vi "Launch Event Handler.vi"(8 "error in (no error)":errorcluster, 11 "Control in":refnum<class "Control.lvclass">) -> (0 "error out":errorcluster, 3 "Control out":refnum<class "Control.lvclass">)   [LabVIEW 2015, in "Control.lvclass"]
doc: "<b> </b> <b> </b>\n©2016 Q Software Innovations, LLC (QSI)\nwritten by Quentin Alldredge\nproduced in LabVIEW 2015\n\nsupport@qsoftwareinnovations.com\nwww.qsoftwareinnovations.com\n\nAll rights reserved.\n\nRedistribution and use in source and binary forms, with or without modification, are permitted provided that the following conditions are met:\n\n * Redistributions of source code must retain the above copyright notice, this list of conditions and the following disclaimer.\n * Redistributions in binary form must reproduce the above copyright notice, this list of conditions and the following disclaimer in the documentation and/or other materials provided with the distribution.\n * Neither the name of Q Software Innovations, LLC. nor the names of its contributors may be used to endorse or promote products derived from this software without specific prior written permission.\n\nTHIS SOFTWARE IS PROVIDED BY THE COPYRIGHT HOLDERS AND CONTRIBUTORS \"AS IS\" AND ANY EXPRESS OR IMPLIED WARRANTIES, INCLUDING, BUT NOT LIMITED TO, THE IMPLIED WARRANTIES OF MERCHANTABILITY AND FITNESS FOR A PARTICULAR PURPOSE ARE DISCLAIMED. IN NO EVENT SHALL THE COPYRIGHT OWNER OR CONTRIBUTORS BE LIABLE FOR ANY DIRECT, INDIRECT, INCIDENTAL, SPECIAL, EXEMPLARY, OR CONSEQUENTIAL DAMAGES (INCLUDING, BUT NOT LIMITED TO, PROCUREMENT OF SUBSTITUTE GOODS OR SERVICES; LOSS OF USE, DATA, OR PROFITS; OR BUSINESS INTERRUPTION) HOWEVER CAUSED AND ON ANY THEORY OF LIABILITY, WHETHER IN CONTRACT, STRICT LIABILITY, OR TORT (INCLUDING NEGLIGENCE OR OTHERWISE) ARISING IN ANY WAY OUT OF THE USE OF THIS SOFTWARE, EVEN IF ADVISED OF THE POSSIBILITY OF SUCH DAMAGE."
uses:
  Control.lvclass
  Control.lvclass/Control.ctl
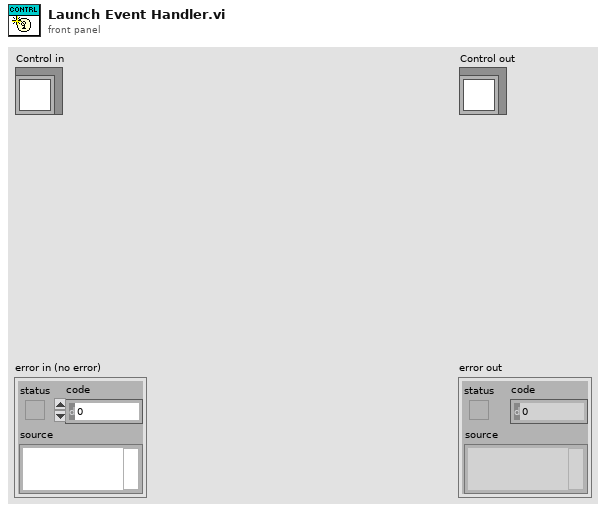
[diagram p1: front panel]
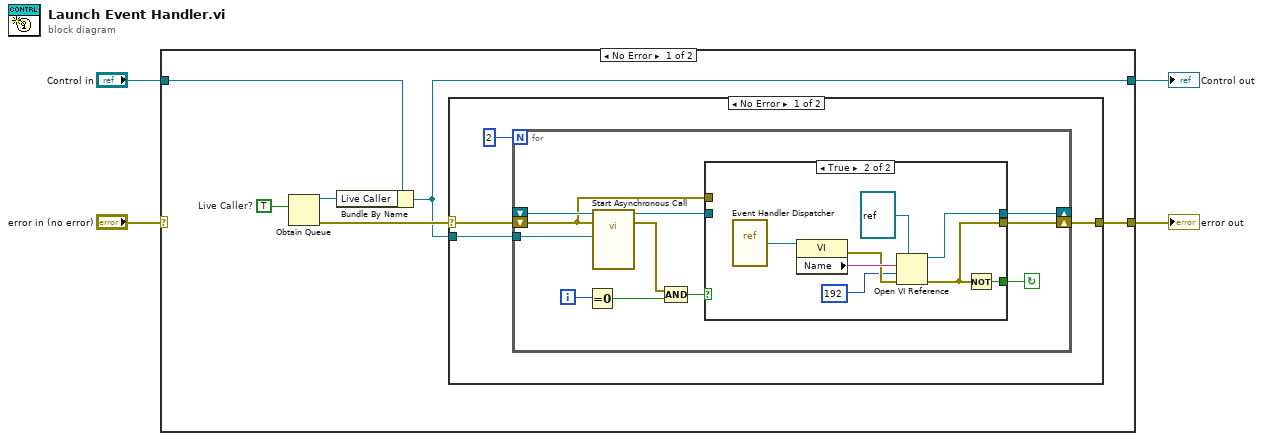
[diagram p0: block diagram]
diagram:
  n1 = case shown="No Error" "error in (no error)" {
    selector: "error in (no error)" -> [_ w38]
    tunnel: [w8 w38] -> w3
    tunnel: [w5 w37] -> w1
    tunnel: "Control in" -> [w6 w37]
    frame No Error {
      w10 = TRUE  # Live Caller?
      n2 = Obtain Queue(element data type=w10) -> (queue out=w7:refnum<queue>, error out=w9:errorcluster)  [unwired: 4 in, 1 out]
      n3 = Bundle By Name(cluster=w6, "Live Caller"=w7) -> (w5:refnum<class "Control.lvclass">)
      n4 = case shown="No Error" w9 {
        selector: w9 -> [w13 w36]
        tunnel: w5 -> [w11 _]
        tunnel: [w12 w36] -> w8
        frame No Error {
          n5 = for {
            N: 2 -> [_]
            tunnel: w11 -> [w25]
            shift-right: [w22] -> _
            shift-left: _ -> [w24]
            shift-right: [w16] -> w12
            shift-left: w13 -> [w15]
            i -> [w20]
            stop <- w21 continue-if-true
            n6 = Equal To 0?(x=w20) -> (x = 0?=w19:bool)
            n7 = call-by-ref "Start Asynchronous Call"(reference=w24, error in=w15, "Control in"=w25) -> (reference out=w23:refnum<vi>, error out=w18:errorcluster)  [unwired: 10 in, 1 out]
            n8 = Compound Arithmetic op=AND(w18, w19) -> (w17:bool)
            n9 = case shown="True" w17 {
              tunnel: w23 -> [w27 _]
              tunnel: [w27 w30] -> w22
              tunnel: [_ w29] -> w21
              tunnel: [w26 w28] -> w16
              tunnel: w15 -> [w26 _]
              frame False {
              }
              frame True {
                n10 = vi-ref "Event Handler Dispatcher.vi"() -> (w35:refnum<vi>)
                n11 = property class="VI"(reference=w35) -> (error out=w33:errorcluster, "Name"=w34:string)  [unwired: 1 in, 1 out]
                n12 = Open VI Reference(type specifier VI Refnum (for type only)=refnum<vi> refnum, vi path=w34, options=192, error in (no error)=w33) -> (vi reference=w30:refnum<vi>, error out=w28:errorcluster)  [unwired: 2 in]
                n13 = Not(x=w28) -> (.not. x?=w29:bool)
              }
            }
          }
        }
        frame Error {
        }
      }
    }
    frame Error {
    }
  }
  "error out" <- w3
  "Control out" <- w1
